vi "read module priority.vi"(7 "Module ID":string, 8 "error in":errorcluster, 11 "Standard Engine Repo Data in":refnum<class "Standard Engine Configuration.lvclass">) -> (0 "error out":errorcluster, 2 "execution order priority":i32, 3 "Standard Engine Repo Data out":refnum<class "Standard Engine Configuration.lvclass">)   [LabVIEW 2013, in "Standard Engine Configuration.lvclass"]
uses:
  Standard Engine Configuration.lvclass
  Standard Engine Configuration.lvclass/Standard Engine Configuration.ctl
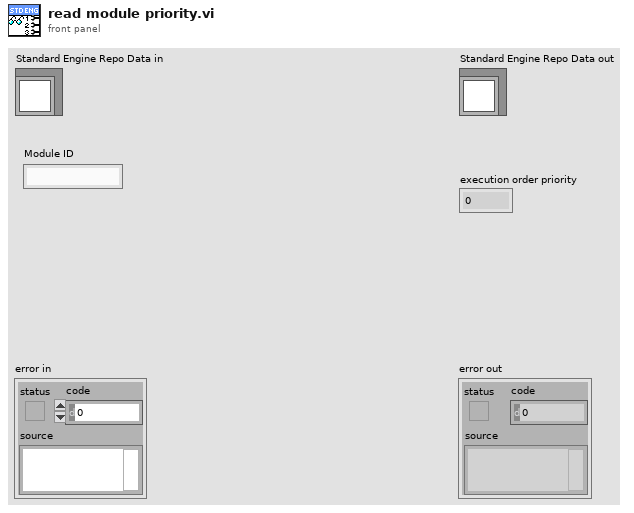
[diagram p1: front panel]
types:
  T1 = typedef "Standard Engine Configuration.lvclass/Module Specific Configuration.ctl" = cluster{"Module ID":string, "Module Decimation":T2, "Module Error Configuration":T3, "execution order priority":i32}
  T2 = typedef "Standard Engine Configuration.lvclass/Module Decimation.ctl" = cluster{"Decimation":u16, "Offset":u16}
  T3 = typedef "Standard Engine Configuration.lvclass/Module Error Configuration.ctl" = cluster{"Module Error Configuration":T4[]}
  T4 = typedef "Standard Engine Configuration.lvclass/Error Actions By Category.ctl" = cluster{"error classification":T5, "Error Actions":T6[]}
  T5 = typedef "TBM module execution interface.lvclass/error classification.ctl" = enum16{"unknown", "none", "trivial", "recoverable", "critical"}
  T6 = typedef "Standard Engine Configuration.lvclass/Error Actions.ctl" = enum16{"Clear", "Notify", "Stop Component", "Stop Engine", "Safe State", "Attempt Recovery"}
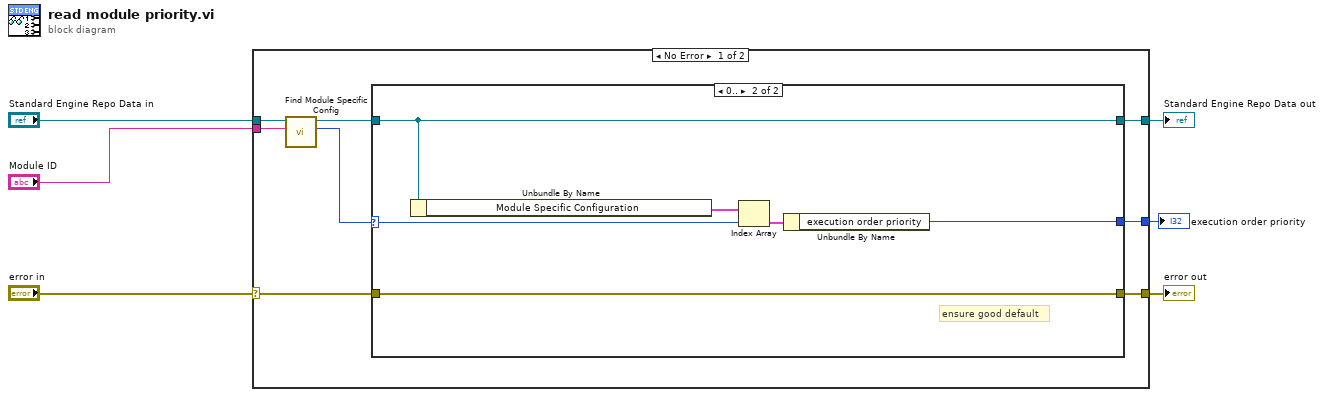
[diagram p0: block diagram]
diagram:
  n1 = case shown="No Error" "error in" {
    selector: "error in" -> [w10 w24]
    tunnel: "Standard Engine Repo Data in" -> [w14 w23]
    tunnel: "Module ID" -> [w13 _]
    tunnel: [w8 w23] -> w4
    tunnel: [w9 w24] -> w2
    tunnel: [w7 _] -> w1
    frame No Error {
      n2 = call "Find Module Specific Config.vi"("Module ID"=w13, "Standard Engine Repo Data in"=w14) -> ("Index"=w11:i32, "Standard Engine Repo Data out"=w12:refnum<class "Standard Engine Configuration.lvclass">)  [unwired: 8 in]
      n3 = case shown="0.." w11 {
        selector: w11 -> [_ w19]
        tunnel: w12 -> [w16 w20]
        tunnel: w10 -> [w15 w18]
        tunnel: [w15 w18] -> w9
        tunnel: [w16 w20] -> w8
        tunnel: [_ w17] -> w7
        frame ..-1 {
        }
        frame 0.. {
          # "ensure good default"
          n4 = Unbundle By Name(w20) -> ("Module Specific Configuration"=w22:T1[])
          n5 = Index Array(array=w22, index=w19) -> (element=w21:T1)
          n6 = Unbundle By Name(w21) -> ("execution order priority"=w17:i32)
        }
      }
    }
    frame Error {
    }
  }
  "error out" <- w2
  "Standard Engine Repo Data out" <- w4
  "execution order priority" <- w1
